vi "Teleop.vi"(10 "Match Info":T1={"Autonomous Elapsed Seconds"=0.0, "TeleOp Elapsed Seconds"=0.0, "Disabled Elapsed Seconds"=0.0, "Visited Autonomous"=FALSE, "Visited TeleOp"=FALSE, "Visited Disabled"=FALSE, "Autonomous Settings"={"Autonomous Style"=enum."Independent", "VI Refnum"=refnum}}, 11 "Call Context":T2) -> ()   [LabVIEW 2017]
doc: "This VI is called for each TeleOp packet received from the DS where the robot is not disabled. It is often used to read from the joysticks and update I/O or to update setpoints for timed control loops. It should complete and return within 20 milliseconds or it may miss DS packets."
uses:
  <vilib>/Rock Robotics/WPI/DriverStation/WPI_DriverStationDerivedRobotMode.ctl
  <vilib>/Rock Robotics/WPI/DriverStation/WPI_DriverStationMatch Info.ctl
  <vilib>/Rock Robotics/WPI/Utilities/WPI_GetSetVariantRefNum.vi
  <vilib>/Rock Robotics/Network Tables/NT Write Boolean Array.vi
  <vilib>/Rock Robotics/Network Tables/NT Write Numeric Array.vi
  <vilib>/Rock Robotics/Network Tables/NT Read Boolean.vi
  <vilib>/Rock Robotics/Network Tables/NT Read Number.vi
  <vilib>/Rock Robotics/Network Tables/NT Read String.vi
  <vilib>/Rock Robotics/Network Tables/NT Write String.vi
panel:
  out "Factor":string
  out "Scale Output":dbl
  out "Sample Slider 0":dbl(slide) scale=0.0..5.0
  out "Sample Boolean 1":bool
  out "Sample Boolean 0":bool
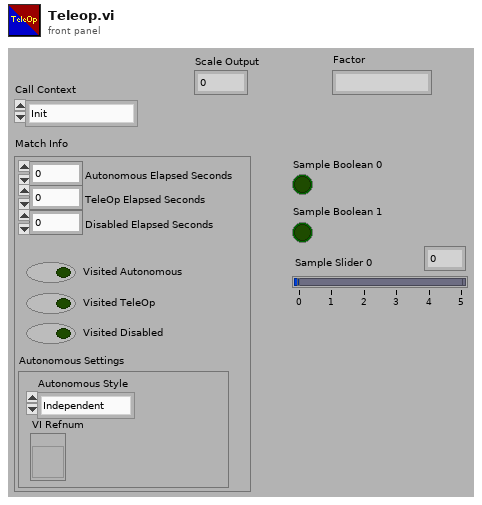
[diagram p1: front panel]
types:
  T1 = typedef "WPI_DriverStationMatch Info.ctl" = cluster{"Autonomous Elapsed Seconds":dbl, "TeleOp Elapsed Seconds":dbl, "Disabled Elapsed Seconds":dbl, "Visited Autonomous":bool, "Visited TeleOp":bool, "Visited Disabled":bool, "Autonomous Settings":cluster{"Autonomous Style":enum16{"Iterative", "Independent"}, "VI Refnum":refnum<vi>}}
  T2 = typedef "WPI_DriverStationDerivedRobotMode.ctl" = enum16{"Init", "Execute", "Stop"}
  T3 = typedef "WPI_RobotDriveDevRef.ctl" = cluster{"DevStatus":errorcluster, "Motors[]":T4[], "Square Inputs":bool, "Max Output":dbl}
  T4 = typedef "WPI_MotorControlDeviceRef.ctl" = cluster{"DeviceStatus":errorcluster, "Type":T5, "PWM":cluster{"PWM Channel":T6, "DeadBand":T7}, "CAN":cluster{"Device Number":u8, "SetOutput VI Ref":variant, "GetOutput VI Ref":variant, "Enable VI Ref":variant, "Disable VI Ref":variant, "Data":variant}, "Invert":bool, "DIO PWM":cluster{"PWM \"Enable\" Channel":T6, "DIOChannel":T8, "PWM Rate":dbl}}
  T5 = typedef "WPI_MotorControlType.ctl" = enum16{"PWM", "CAN", "DIO PWM"}
  T6 = typedef "FPGA_DIOPWMChannel.ctl" = enum8{"PWM 0", "PWM 1", "PWM 2", "PWM 3", "PWM 4", "PWM 5", "PWM 6", "PWM 7", "PWM 8", "PWM 9", "PWM MXP 0", "PWM MXP 1", "PWM MXP 2", "PWM MXP 3", "PWM MXP 4", "PWM MXP 5", "PWM MXP 6", "PWM MXP 7", "PWM MXP 8", "PWM MXP 9", "Invalid"}
  T7 = typedef "WPI_PWMDeadband.ctl" = cluster{"Name":string, "maxPositivePwm":i32, "minPositivePwm":i32, "centerPwm":i32, "maxNegativePwm":i32, "minNegativePwm":i32, "angularRange":u16}
  T8 = typedef "FPGA_DIOChannel.ctl" = enum8{"DIO 0", "DIO 1", "DIO 2", "DIO 3", "DIO 4", "DIO 5", "DIO 6", "DIO 7", "DIO 8", "DIO 9", "DIO MXP 0", "DIO MXP 1", "DIO MXP 2", "DIO MXP 3", "DIO MXP 4", "DIO MXP 5", "DIO MXP 6", "DIO MXP 7", "DIO MXP 8", "DIO MXP 9", "DIO MXP 10", "DIO MXP 11", "DIO MXP 12", "DIO MXP 13", "DIO MXP 14", "DIO MXP 15", "SPI Port CS1", "SPI Port CS2", "SPI Port CS3", "SPI Port MISO", "SPI Port MOSI", "Invalid"}
  T9 = typedef "WPI_JoystickDevRef.ctl" = cluster{"Device":T10}
  T10 = typedef "WPI_JoystickDeviceEnum.ctl" = enum16{"USB 0", "USB 1", "USB 2", "USB 3", "USB 4", "USB 5"}
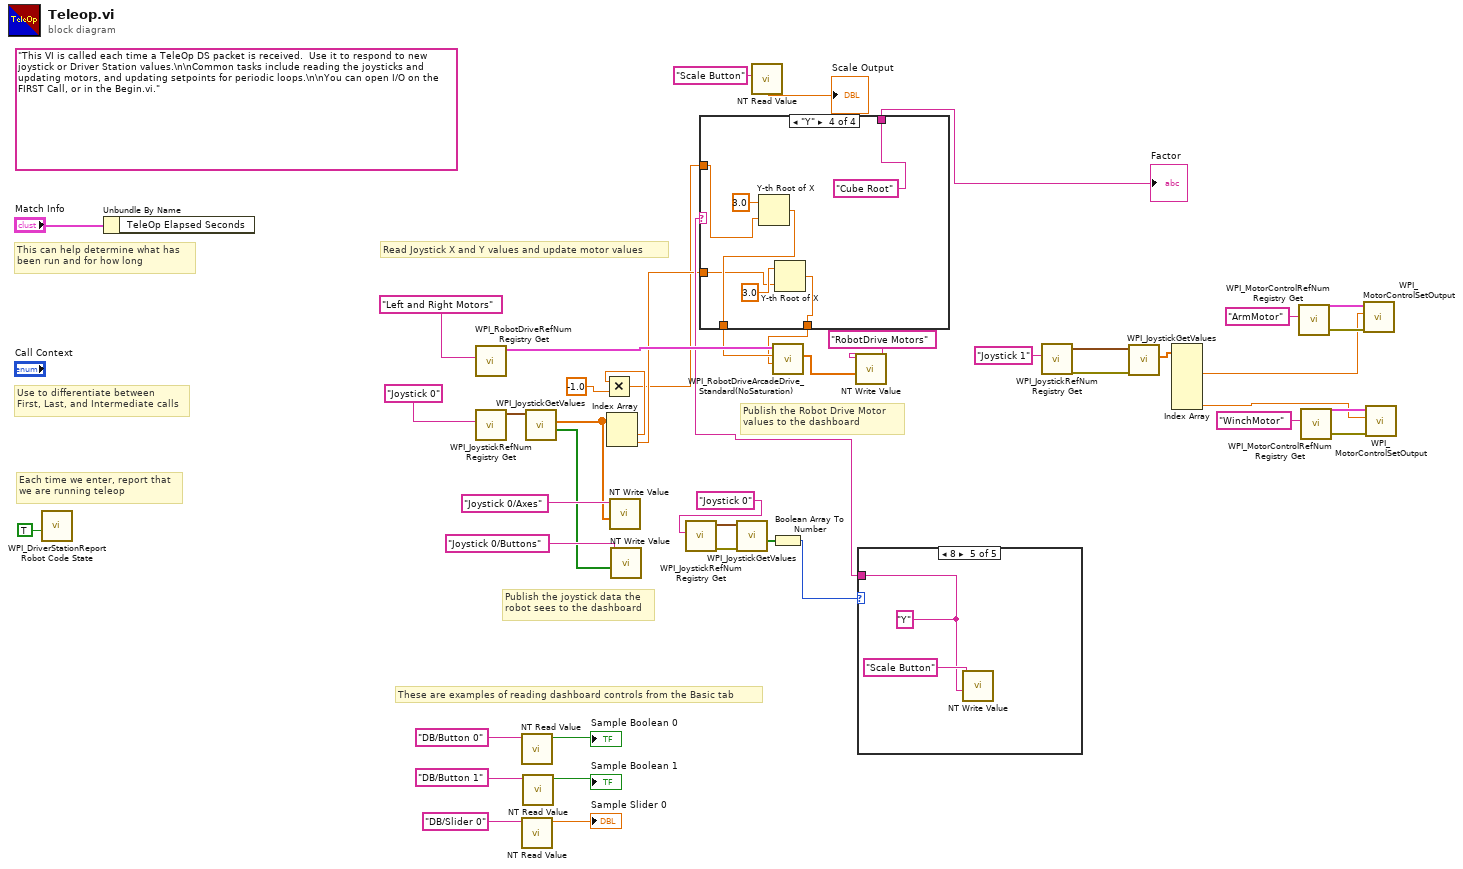
[diagram p0: block diagram]
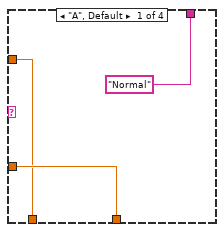
[diagram p2: hidden frame]
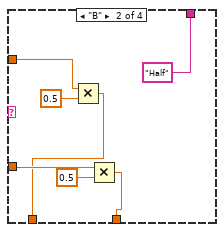
[diagram p3: hidden frame]
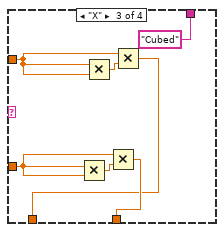
[diagram p4: hidden frame]
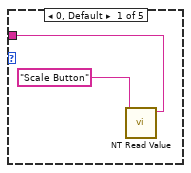
[diagram p5: hidden frame]
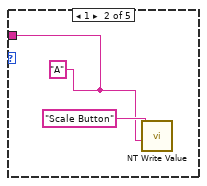
[diagram p6: hidden frame]
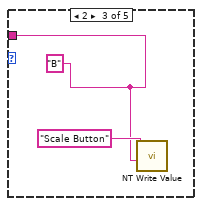
[diagram p7: hidden frame]
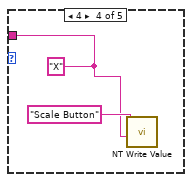
[diagram p8: hidden frame]
diagram:
  (unwired) "This VI is called each time a TeleOp DS packet is received.  Use it to respond to new joystick or Driver Station values.\n\nCommon tasks include reading the joysticks and updating motors, and updating setpoints for periodic loops.\n\nYou can open I/O on the FIRST Call, or in the Begin.vi."
  # "These are examples of reading dashboard controls from the Basic tab"
  # "Publish the Robot Drive Motor\nvalues to the dashboard"
  # "Publish the joystick data the\nrobot sees to the dashboard"
  # "Each time we enter, report that\nwe are running teleop"
  # "Use to differentiate between\nFirst, Last, and Intermediate calls"
  # "This can help determine what has\nbeen run and for how long"
  # "Read Joystick X and Y values and update motor values"
  n1 = call <vilib>:"WPI_DriverStationReport Robot Code State.vi"("TeleOp"=TRUE ("Autonomous")) -> ()  [unwired: 10 in, 1 out]
  n2 = Unbundle By Name("Match Info") -> ()  [unwired: 1 out]
  n3 = call <vilib>:"WPI_RobotDriveRefNum Registry Get.vi"("refnum name"="Left and Right Motors") -> ("RobotDriveDevRef"=w43:T3)  [unwired: 1 in, 9 out]
  n4 = call <vilib>:"WPI_JoystickRefNum Registry Get.vi"("refnum name"="Joystick 0") -> ("JoystickDevRef"=w41:T9)  [unwired: 1 in, 9 out]
  n5 = call-poly <vilib>:"NT Read Value.vi"("Name"="DB/Button 0" ("refnum name")) -> ("Boolean"=→"Sample Boolean 0":bool)  [unwired: 9 in, 1 out]
  n6 = call-poly <vilib>:"NT Read Value.vi"("Name"="DB/Slider 0" ("refnum name")) -> ("Numeric"=→"Sample Slider 0":dbl)  [unwired: 9 in, 1 out]
  n7 = call-poly <vilib>:"NT Read Value.vi"("Name"="DB/Button 1" ("refnum name")) -> ("Boolean"=→"Sample Boolean 1":bool)  [unwired: 9 in, 1 out]
  n8 = call <vilib>:"WPI_JoystickGetValues.vi"("JoystickDevRef"=w41) -> ("Buttons"=w29:bool[], "Axes"=w30:dbl[])  [unwired: 6 in, 3 out]
  n9 = Index Array(array=w30) -> (element #1=w2:dbl, element #2=w3:dbl)  [unwired: 2 in]
  n10 = Multiply(x=w2, y=-1.0) -> (x*y=w1:dbl)
  n11 = call-poly <vilib>:"NT Write Value.vi"("Numeric Array"=w30, "Name"="Joystick 0/Axes") -> ()  [unwired: 9 in, 1 out]
  n12 = call-poly <vilib>:"NT Write Value.vi"("Boolean Array"=w29, "Name"="Joystick 0/Buttons") -> ()  [unwired: 9 in, 1 out]
  n13 = call <vilib>:"WPI_JoystickRefNum Registry Get.vi"("refnum name"="Joystick 0") -> ("error out"=w27:errorcluster, "JoystickDevRef"=w26:T9)  [unwired: 9 in]
  n14 = call <vilib>:"WPI_JoystickGetValues.vi"("error in (no error)"=w27, "JoystickDevRef"=w26) -> ("Buttons"=w28:bool[])  [unwired: 5 in, 4 out]
  n15 = call-poly <vilib>:"NT Read Value.vi"("Name"="Scale Button") -> ("Numeric"=→"Scale Output":dbl)  [unwired: 9 in, 1 out]
  n16 = Boolean Array To Number(Boolean array=w28) -> (number=w22:u32)
  n17 = case shown="8" w22 {
    tunnel: [w46 w48 w50 w52 w54] -> w21
    frame 0, Default {
      n18 = call-poly <vilib>:"NT Read Value.vi"("Name"="Scale Button") -> ("String"=w46:string)  [unwired: 9 in, 1 out]
    }
    frame 1 {
      w48 = "A"
      n19 = call-poly <vilib>:"NT Write Value.vi"("String"=w48, "Name"="Scale Button") -> ()  [unwired: 9 in, 1 out]
    }
    frame 2 {
      w50 = "B"
      n20 = call-poly <vilib>:"NT Write Value.vi"("String"=w50, "Name"="Scale Button") -> ()  [unwired: 9 in, 1 out]
    }
    frame 4 {
      w52 = "X"
      n21 = call-poly <vilib>:"NT Write Value.vi"("String"=w52, "Name"="Scale Button") -> ()  [unwired: 9 in, 1 out]
    }
    frame 8 {
      w54 = "Y"
      n22 = call-poly <vilib>:"NT Write Value.vi"("String"=w54, "Name"="Scale Button") -> ()  [unwired: 9 in, 1 out]
    }
  }
  n23 = case shown="\"Y\"" w21 {
    tunnel: w1 -> [w56 w64 w70 w76]
    tunnel: ["Normal" "Half" "Cubed" "Cube Root"] -> w20
    tunnel: w3 -> [w57 w61 w68 w73]
    tunnel: [w57 w59 w67 w78] -> w5
    tunnel: [w56 w60 w66 w77] -> w18
    frame "A", Default {
    }
    frame "B" {
      n24 = Multiply(x=w64, y=0.5) -> (x*y=w60:dbl)
      n25 = Multiply(x=w61, y=0.5) -> (x*y=w59:dbl)
    }
    frame "X" {
      n26 = Multiply(x=w68, y=w68) -> (x*y=w69:dbl)
      n27 = Multiply(x=w70, y=w70) -> (x*y=w72:dbl)
      n28 = Multiply(x=w68, y=w69) -> (x*y=w67:dbl)
      n29 = Multiply(x=w70, y=w72) -> (x*y=w66:dbl)
    }
    frame "Y" {
      n30 = Y-th Root of X(1:w76, 2:3.0 ("y")) -> (0:w77:dbl)
      n31 = Y-th Root of X(1:w73, 2:3.0) -> (0:w78:dbl)
    }
  }
  "Factor" <- w20
  n32 = call <vilib>:"WPI_RobotDriveArcadeDrive_Standard(NoSaturation).vi"("Y axis value"=w5, "X axis value"=w18, "RobotDriveDevRef"=w43) -> ("Motor Values"=w19:dbl[])  [unwired: 1 in, 7 out]
  n33 = call-poly <vilib>:"NT Write Value.vi"("Numeric Array"=w19, "Name"="RobotDrive Motors") -> ()  [unwired: 9 in, 1 out]
  n34 = call <vilib>:"WPI_JoystickRefNum Registry Get.vi"("refnum name"="Joystick 1") -> ("error out"=w16:errorcluster, "JoystickDevRef"=w17:T9)  [unwired: 9 in]
  n35 = call <vilib>:"WPI_JoystickGetValues.vi"("error in (no error)"=w16, "JoystickDevRef"=w17) -> ("Axes"=w14:dbl[])  [unwired: 5 in, 4 out]
  n36 = Index Array(array=w14) -> (element #2=w7:dbl, element #6=w6:dbl)  [unwired: 6 in, 4 out]
  n37 = call <vilib>:"WPI_MotorControlRefNum Registry Get.vi"("refnum name"="ArmMotor") -> ("error out"=w12:errorcluster, "MotorControlDevRef"=w13:T4)  [unwired: 9 in]
  n38 = call <vilib>:"WPI_MotorControlRefNum Registry Get.vi"("refnum name"="WinchMotor") -> ("error out"=w9:errorcluster, "MotorControlDevRef"=w10:T4)  [unwired: 9 in]
  n39 = call <vilib>:"WPI_MotorControlSetOutput.vi"("error in (no error)"=w12, "Output"=w7, "MotorControlDevRef"=w13) -> ()  [unwired: 6 in, 3 out]
  n40 = call <vilib>:"WPI_MotorControlSetOutput.vi"("error in (no error)"=w9, "Output"=w6, "MotorControlDevRef"=w10) -> ()  [unwired: 6 in, 3 out]
